vi "server.vi"() -> ()   [LabVIEW 2019]
uses:
  <vilib>/NI/NI JSONRPC Server Framework/Classes/Request/Request.lvclass/Request.ctl
  <vilib>/NI/NI JSONRPC Server Framework/Classes/Request/request.Read method.vi
  <vilib>/NI/NI JSONRPC Server Framework/Classes/Request/request.Read params.vi
  <vilib>/NI/NI JSONRPC Server Framework/Classes/params/params.To JSON Tree.vi
  <vilib>/NI/NI JSONRPC Server Framework/Classes/Server/Add Response (Result from Request).vi
  <vilib>/NI/NI JSONRPC Server Framework/Classes/Server/Add Response (Server Error from Request).vi
  <vilib>/NI/NI JSONRPC Server Framework/Classes/Server/Add Response (Internal Error from Request).vi
  <vilib>/NI/NI JSONRPC Server Framework/Classes/Server/Send Request (Sync).vi
  <vilib>/NI/JSON Support for LabVIEW/JSON Value/JSON Value.lvclass
  <vilib>/NI/NI JSONRPC Server Framework/Classes/Server/JSONRPC Server.lvclass
  <vilib>/NI/NI JSONRPC Server Framework/Classes/Request/Request.lvclass
panel:
  out "Input JSON Strings":string
  out "Output Data Array":dbl[][](array[numeric])
  out "Output JSON Strings":string
  out "Response String Length":i32
  in  "stop server":bool
  # "Input Data"
  # "Output Data"
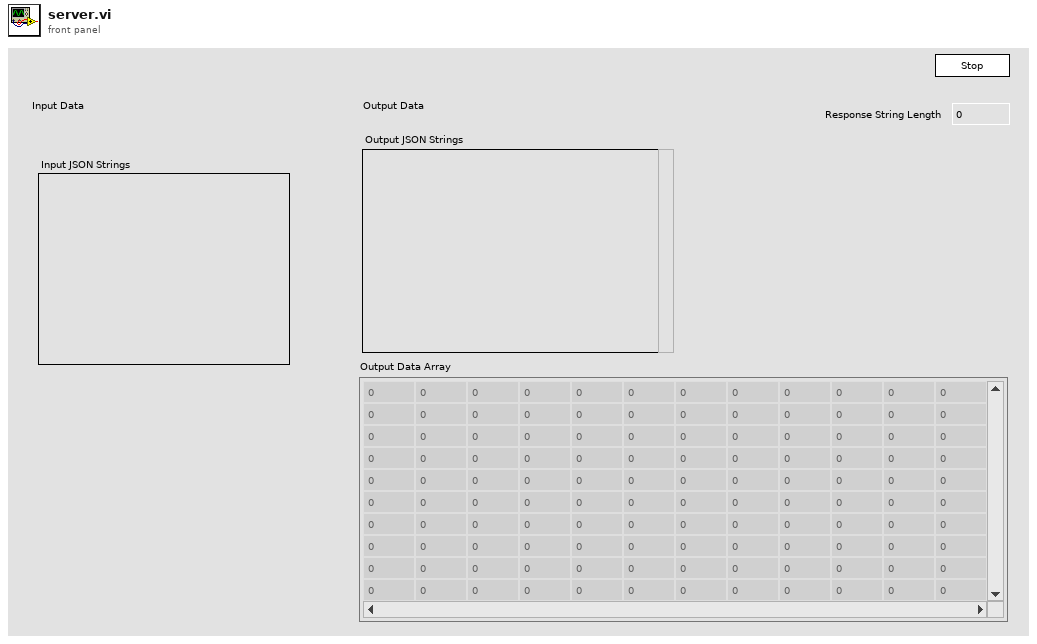
[diagram p1: front panel]
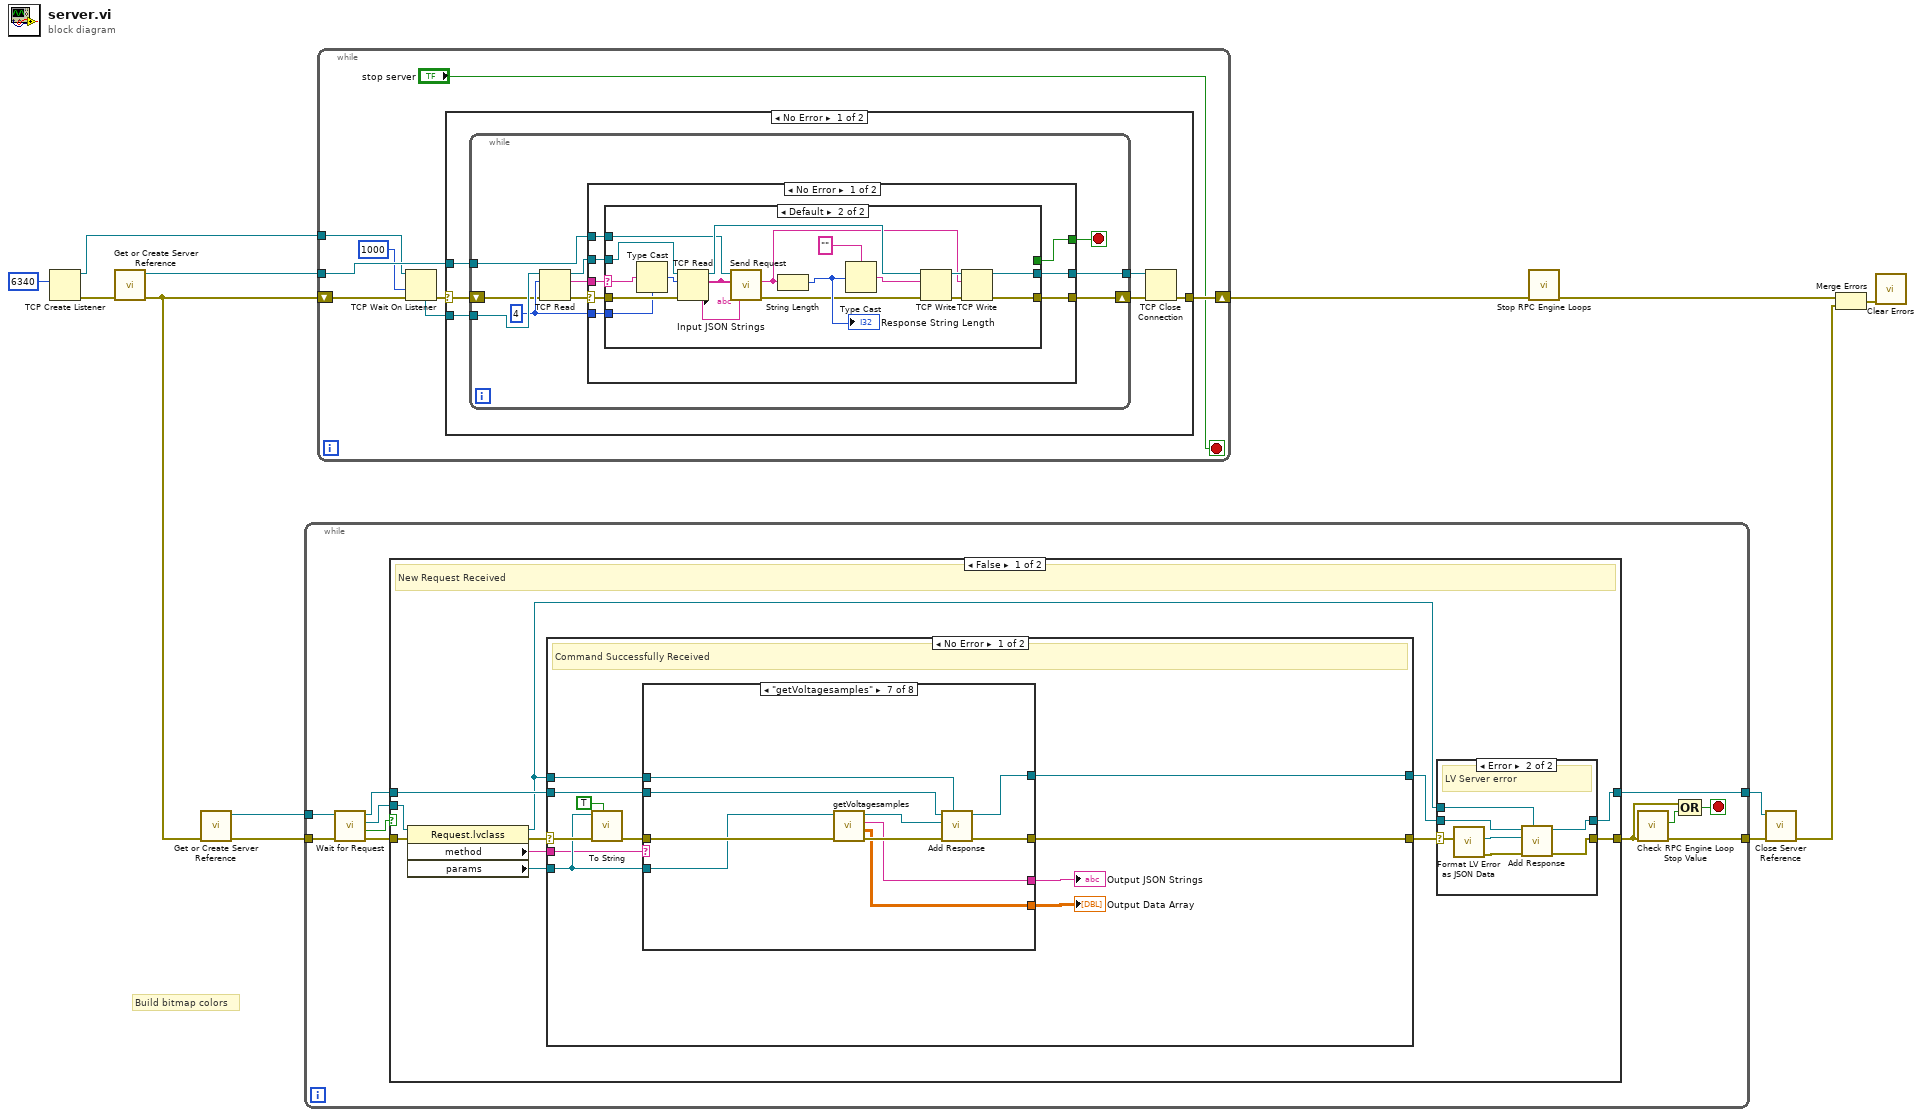
[diagram p0: block diagram]
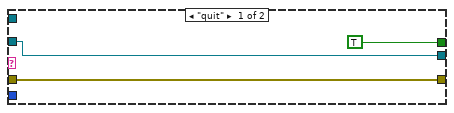
[diagram p2: hidden frame]
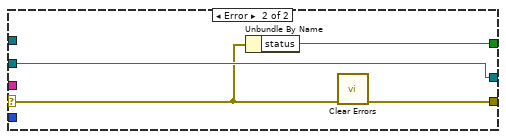
[diagram p3: hidden frame]
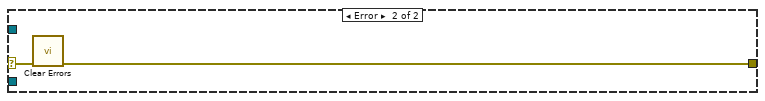
[diagram p4: hidden frame]
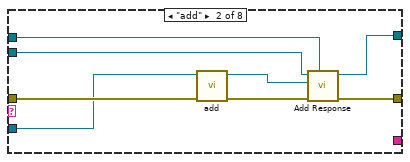
[diagram p6: hidden frame]
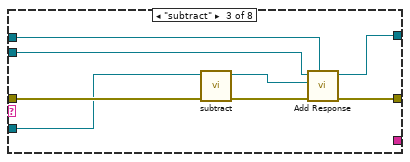
[diagram p7: hidden frame]
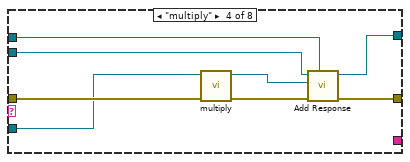
[diagram p8: hidden frame]
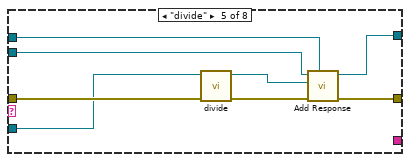
[diagram p9: hidden frame]
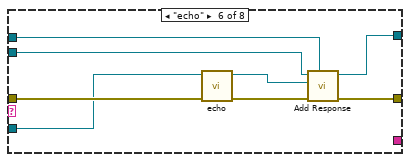
[diagram p10: hidden frame]
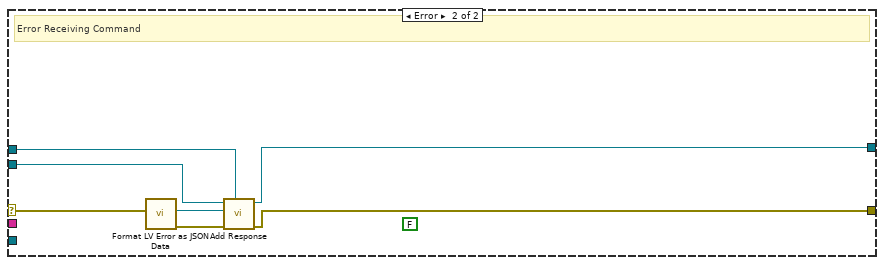
[diagram p12: hidden frame]
diagram:
  # "Build bitmap colors"
  n1 = TCP Create Listener(10:u16 6340 ("remote port or service name")) -> (0:w8:errorcluster, 3:w10:refnum<k5>)  [unwired: 4 in, 1 out]
  n2 = call <vilib>:"Get or Create Server Reference.vi"("error in (no error)"=w8) -> ("error out"=w2:errorcluster, "Server Out"=w13:refnum<class "JSONRPC Server.lvclass">)  [unwired: 9 in]
  n3 = call <vilib>:"Get or Create Server Reference.vi"("error in (no error)"=w2) -> ("error out"=w4:errorcluster, "Server Out"=w3:refnum<class "JSONRPC Server.lvclass">)  [unwired: 9 in]
  n4 = while {
    tunnel: w3 -> [w24]
    tunnel: w4 -> [w20]
    tunnel: [w15] -> w6
    tunnel: [w18] -> w5
    stop <- w17 stop-if-true
    n5 = call <vilib>:"Wait for Request.vi"("error in (no error)"=w20, "Server in"=w24) -> ("error out"=w19:errorcluster, "timed out?"=w21:bool, "Request"=w22:refnum<class "Request.lvclass">, "Server out"=w23:refnum<class "JSONRPC Server.lvclass">)  [unwired: 6 in]
    n6 = case shown="False" w21 {
      tunnel: w23 -> [w30 w117]
      tunnel: w22 -> [w35 _]
      tunnel: w19 -> [w32 w118]
      tunnel: [w28 w118] -> w16
      tunnel: [w26 w117] -> w18
      frame False {
        # "New Request Received"
        n7 = property class="Request.lvclass"(reference=w35, error in=w32) -> (reference out=w25:refnum<class "Request.lvclass">, error out=w31:errorcluster, "method"=w34:string, "params"=w33:refnum<class "JSON Value.lvclass">)
        n8 = case shown="No Error" w31 {
          selector: w31 -> [w43 w102]
          tunnel: w34 -> [w38 _]
          tunnel: w33 -> [w41 _]
          tunnel: [w39 w104] -> w29
          tunnel: w30 -> [w46 w106]
          tunnel: [w45 w105] -> w27
          tunnel: w25 -> [w44 w107]
          frame No Error {
            # "Command Successfully Received"
            n9 = call <vilib>:"To String.vi"("pretty print? (F)"=TRUE, "error in (no error)"=w43, "JSON Value in"=w41) -> ("error out"=w42:errorcluster)  [unwired: 7 in, 1 out]
            n10 = case shown="\"getVoltagesamples\"" w38 {
              tunnel: w42 -> [w48 w56 w60 w68 w76 w84 w94 w100]
              tunnel: w46 -> [w47 w51 w62 w70 w78 w86 w96 w99]
              tunnel: [w48 w53 w64 w72 w80 w88 w98 w100] -> w39
              tunnel: [w47 w52 w63 w71 w79 w87 w97 w99] -> w45
              tunnel: w44 -> [_ w49 w61 w69 w77 w85 w95 _]
              tunnel: w41 -> [_ w55 w59 w65 w73 w81 w93 _]
              tunnel: [_ _ _ _ _ _ w89 _] -> w37
              tunnel: [_ _ _ _ _ _ w90 _] -> w36
              frame Default {
              }
              frame "add" {
                n11 = call "add.vi"("error in (no error)"=w56, "params"=w55) -> ("error out"=w54:errorcluster, "data"=w50:refnum<class "JSON Value.lvclass">)  [unwired: 8 in]
                n12 = call-poly <vilib>:"Add Response.vi"("Request"=w49, "error in (no error)"=w54, "JSON Value in"=w50, "Server in"=w51) -> ("error out"=w53:errorcluster, "Server out"=w52:refnum<class "JSONRPC Server.lvclass">)  [unwired: 5 in, 1 out]
              }
              frame "subtract" {
                n13 = call "subtract.vi"("error in (no error)"=w60, "params"=w59) -> ("error out"=w57:errorcluster, "data"=w58:refnum<class "JSON Value.lvclass">)  [unwired: 8 in]
                n14 = call-poly <vilib>:"Add Response.vi"("Request"=w61, "error in (no error)"=w57, "JSON Value in"=w58, "Server in"=w62) -> ("error out"=w64:errorcluster, "Server out"=w63:refnum<class "JSONRPC Server.lvclass">)  [unwired: 5 in, 1 out]
              }
              frame "multiply" {
                n15 = call "multiply.vi"("error in (no error)"=w68, "params"=w65) -> ("error out"=w67:errorcluster, "data"=w66:refnum<class "JSON Value.lvclass">)  [unwired: 8 in]
                n16 = call-poly <vilib>:"Add Response.vi"("Request"=w69, "error in (no error)"=w67, "JSON Value in"=w66, "Server in"=w70) -> ("error out"=w72:errorcluster, "Server out"=w71:refnum<class "JSONRPC Server.lvclass">)  [unwired: 5 in, 1 out]
              }
              frame "divide" {
                n17 = call "divide.vi"("error in (no error)"=w76, "params"=w73) -> ("error out"=w75:errorcluster, "data"=w74:refnum<class "JSON Value.lvclass">)  [unwired: 8 in]
                n18 = call-poly <vilib>:"Add Response.vi"("Request"=w77, "error in (no error)"=w75, "JSON Value in"=w74, "Server in"=w78) -> ("error out"=w80:errorcluster, "Server out"=w79:refnum<class "JSONRPC Server.lvclass">)  [unwired: 5 in, 1 out]
              }
              frame "echo" {
                n19 = call "echo.vi"("error in (no error)"=w84, "params"=w81) -> ("error out"=w83:errorcluster, "data"=w82:refnum<class "JSON Value.lvclass">)  [unwired: 8 in]
                n20 = call-poly <vilib>:"Add Response.vi"("Request"=w85, "error in (no error)"=w83, "JSON Value in"=w82, "Server in"=w86) -> ("error out"=w88:errorcluster, "Server out"=w87:refnum<class "JSONRPC Server.lvclass">)  [unwired: 5 in, 1 out]
              }
              frame "getVoltagesamples" {
                n21 = call "getVoltagesamples.vi"("error in (no error)"=w94, "params"=w93) -> ("error out"=w91:errorcluster, "Voltage Samples"=w90:dbl[][], "JSON String"=w89:string, "data"=w92:refnum<class "JSON Value.lvclass">)  [unwired: 6 in]
                n22 = call-poly <vilib>:"Add Response.vi"("Request"=w95, "error in (no error)"=w91, "JSON Value in"=w92, "Server in"=w96) -> ("error out"=w98:errorcluster, "Server out"=w97:refnum<class "JSONRPC Server.lvclass">)  [unwired: 5 in, 1 out]
              }
              frame "shutdown_rpc_server" {
              }
            }
            "Output JSON Strings" <- w37
            "Output Data Array" <- w36
          }
          frame Error {
            (unwired) FALSE
            # "Error Receiving Command"
            n23 = call <vilib>:"Format LV Error as JSON Data.vi"("error in"=w102) -> ("error out"=w103:errorcluster, "Error Value out"=w101:refnum<class "JSON Value.lvclass">)  [unwired: 9 in]
            n24 = call-poly <vilib>:"Add Response.vi"("Request"=w107, "error in (no error)"=w103, "data"=w101, "Server in"=w106) -> ("error out"=w104:errorcluster, "Server out"=w105:refnum<class "JSONRPC Server.lvclass">)  [unwired: 5 in, 1 out]
          }
        }
        n25 = case shown="Error" w29 {
          selector: w29 -> [w109 w112]
          tunnel: [w109 w111] -> w28
          tunnel: w27 -> [w108 w115]
          tunnel: [w108 w114] -> w26
          tunnel: w25 -> [_ w110]
          frame No Error {
          }
          frame Error {
            # "LV Server error"
            n26 = call <vilib>:"Format LV Error as JSON Data.vi"("error in"=w112) -> ("error out"=w113:errorcluster, "Error Value out"=w116:refnum<class "JSON Value.lvclass">)  [unwired: 9 in]
            n27 = call-poly <vilib>:"Add Response.vi"("Request"=w110, "error in (no error)"=w113, "data"=w116, "Server in"=w115) -> ("error out"=w111:errorcluster, "Server out"=w114:refnum<class "JSONRPC Server.lvclass">)  [unwired: 5 in, 1 out]
          }
        }
      }
      frame True {
        # "Timeout while waiting for new Requests"
      }
    }
    n28 = call <vilib>:"Check RPC Engine Loop Stop Value.vi"("error in (no error)"=w16) -> ("error out"=w15:errorcluster, "stopped?"=w14:bool)  [unwired: 9 in]
    n29 = Compound Arithmetic op=OR(w16, w14) -> (w17:bool)
  }
  n30 = while {
    tunnel: w13 -> [w126]
    tunnel: w10 -> [w124]
    shift-right: [w125] -> w12
    shift-left: w2 -> [w122]
    stop <- "stop server" stop-if-true
    n31 = TCP Wait On Listener(8:w122, 9:1000 ("timeout ms (wait forever: -1)"), 11:w124) -> (0:w121:errorcluster, 4:w123:refnum<k5>)  [unwired: 1 in, 3 out]
    n32 = case shown="No Error" w121 {
      selector: w121 -> [w127 w177]
      tunnel: w126 -> [w132 _]
      tunnel: [w131 w176] -> w125
      tunnel: w123 -> [w128 _]
      frame No Error {
        n33 = while {
          tunnel: w132 -> [w142]
          shift-right: [w134] -> w130
          shift-left: w127 -> [w135]
          tunnel: [w141] -> w129
          tunnel: w128 -> [w140]
          stop <- w133 stop-if-true
          w137 = 4 ("bytes to read")
          n34 = TCP Read(connection ID=w140, bytes to read=w137, error in (no error)=w135) -> (connection ID out=w138:refnum<k5>, data out=w139:string, error out=w136:errorcluster)  [unwired: 2 in]
          n35 = case shown="No Error" w136 {
            selector: w136 -> [w150 w173]
            tunnel: w139 -> [w149 _]
            tunnel: w138 -> [w148 w174]
            tunnel: [w147 w174] -> w141
            tunnel: [w146 w175] -> w134
            tunnel: w137 -> [w145 _]
            tunnel: w142 -> [w144 _]
            tunnel: [w143 w172] -> w133
            frame No Error {
              n36 = case shown="Default" w149 {
                selector: w149 -> [_ w170]
                tunnel: w150 -> [w153 w171]
                tunnel: w148 -> [w152 w169]
                tunnel: [w152 w168] -> w147
                tunnel: [w153 w167] -> w146
                tunnel: w145 -> [_ w159]
                tunnel: w144 -> [_ w155]
                tunnel: [TRUE _] -> w143
                frame "quit" {
                }
                frame Default {
                  n37 = Type Cast(type=w159, x=w170) -> (*(type *) &x=w160:i32)
                  n38 = TCP Read(connection ID=w169, bytes to read=w160, error in (no error)=w171) -> (connection ID out=w164:refnum<k5>, data out=w154:string, error out=w158:errorcluster)  [unwired: 2 in]
                  "Input JSON Strings" <- w154
                  n39 = call-poly <vilib>:"Send Request.vi"("error in (no error)"=w158, "JSON Request String"=w154, "JSONRPC Server in"=w155) -> ("error out"=w157:errorcluster, "JSON Response String"=w156:string)  [unwired: 6 in, 1 out]
                  n40 = String Length(string=w156) -> (length=w163:i32)
                  "Response String Length" <- w163
                  n41 = Type Cast(type="", x=w163) -> (*(type *) &x=w161:string)
                  n42 = TCP Write(connection ID=w164, data in=w161, error in (no error)=w157) -> (connection ID out=w165:refnum<k5>, error out=w166:errorcluster)  [unwired: 1 in, 1 out]
                  n43 = TCP Write(connection ID=w165, data in=w156, error in (no error)=w166) -> (connection ID out=w168:refnum<k5>, error out=w167:errorcluster)  [unwired: 1 in, 1 out]
                }
              }
            }
            frame Error {
              n44 = Unbundle By Name(w173) -> ("status"=w172:bool)
              n45 = call <vilib>:"Clear Errors.vi"("error in (no error)"=w173) -> ("error out"=w175:errorcluster)  [unwired: 5 in, 1 out]
            }
          }
        }
        n46 = TCP Close Connection(connection ID=w129, error in (no error)=w130) -> (error out=w131:errorcluster)  [unwired: 1 in, 1 out]
      }
      frame Error {
        n47 = call <vilib>:"Clear Errors.vi"("error in (no error)"=w177) -> ("error out"=w176:errorcluster)  [unwired: 5 in, 1 out]
      }
    }
  }
  n48 = call <vilib>:"Stop RPC Engine Loops.vi"("error in (no error)"=w12) -> ("error out"=w9:errorcluster)  [unwired: 10 in]
  n49 = call <vilib>:"Close Server Reference.vi"("error in (no error)"=w6, "Server in"=w5) -> ("error out"=w1:errorcluster)  [unwired: 9 in]
  n50 = Merge Errors(w9, w1) -> (w7:errorcluster)
  n51 = call <vilib>:"Clear Errors.vi"("error in (no error)"=w7) -> ()  [unwired: 5 in, 2 out]
